vi "ButtonToggle.vi"(1 "Button":bool) -> (0 "Value":bool)   [LabVIEW 2014]
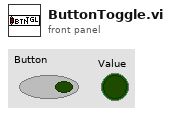
[diagram p1: front panel]
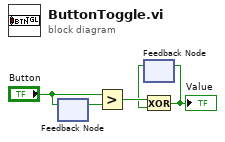
[diagram p0: block diagram]
diagram:
  n1 = feedback #1() -> (w5:bool)  [unwired: 1 in]
  n2 = feedback-in #1("Button") -> ()
  n3 = Greater?(x="Button", y=w5) -> (0:w3:bool)
  n4 = feedback #2() -> (w2:bool)  [unwired: 1 in]
  n5 = Exclusive Or(1:w2, 2:w3) -> (0:w1:bool)
  "Value" <- w1
  n6 = feedback-in #2(w1) -> ()
